vi "Decoding 4-point FPGA Values.vi"(1 "DMA Data":u64[](array[numeric])=[1, 2, 3, 4] format="%.0b") -> (0 "[I16] All points in correct chronological order":i16[](array[numeric]))   [LabVIEW 2017]
panel:
  # "Oldest point"
  # "Oldest point"
  # "Oldest point"
  # "Newest point"
  # "Newest point"
  # "Oldest point"
  # "Newest point"
  # "Oldest point"
  # "Newest point"
  # "Oldest point"
  # "Newest point"
  # "Newest point"
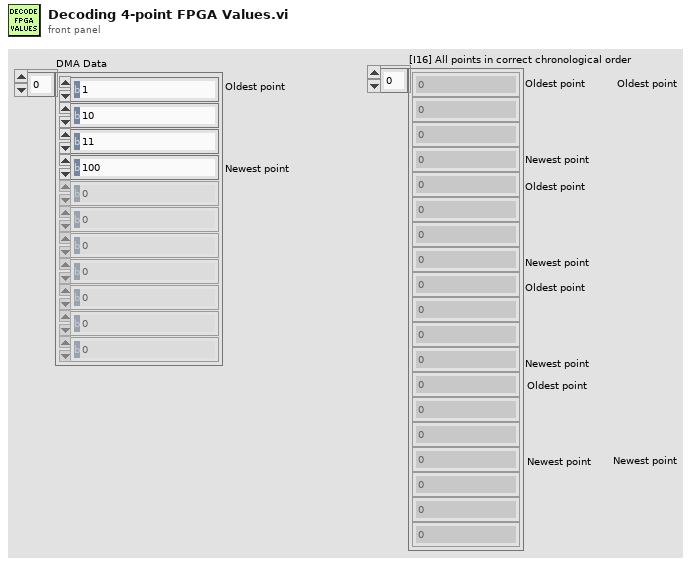
[diagram p1: front panel]
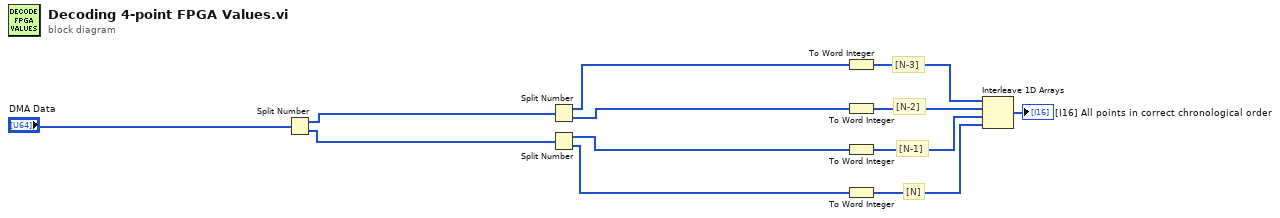
[diagram p0: block diagram]
diagram:
  # "[N-3]"
  # "[N-2]"
  # "[N-1]"
  # "[N]"
  n1 = Split Number(x="DMA Data") -> (hi(x)=w12:u32[], lo(x)=w9:u32[])
  n2 = Split Number(x=w12) -> (hi(x)=w11:u16[], lo(x)=w10:u16[])
  n3 = Split Number(x=w9) -> (hi(x)=w8:u16[], lo(x)=w7:u16[])
  n4 = To Word Integer(number=w11) -> (16bit integer=w5:i16[])
  n5 = To Word Integer(number=w10) -> (16bit integer=w4:i16[])
  n6 = To Word Integer(number=w8) -> (16bit integer=w3:i16[])
  n7 = To Word Integer(number=w7) -> (16bit integer=w2:i16[])
  n8 = Interleave 1D Arrays "Interleave 1D Arrays"(w5, w4, w3, w2) -> (→"[I16] All points in correct chronological order":i16[])
